vi "main(Test DQMH modules).bak.vi"() -> ()   [LabVIEW 2018, in "Application.lvlib"] (continued)
              frame Disabled {
              }
            }
          }
          event "Test Channel 1": Value Change {
            n428 = event-data() -> ()  [unwired: 1 in, 1 out]
            n429 = Array Subset(array=w1027, index=0, length=6) -> (w1024:refnum<vi>[])
            n430 = for {
              tunnel: w1024 -> [w1036] mode=indexing
              n431 = property class="ColBox"(reference=w1036, "Value"=u32 10000536 ("DRV 1")) -> ()  [unwired: 1 in, 2 out]
            }
            n432 = Build Array("Test Channel 1", "MEAS.AllRelaysOFF") -> (w1031:string[])
            n433 = for {
              tunnel: [w1040] -> w1032 mode=indexing
              tunnel: w1031 -> [w1039] mode=indexing
              tunnel: w1030 -> [w1038]
              n434 = call "App enquece.vi"("command"=w1039, "queue in"=w1038) -> ("error out"=w1040:errorcluster)  [unwired: 8 in, 1 out]
            }
            n435 = Merge Errors(w1034, w1032) -> (w1033:errorcluster)
          }
          event "Test Channel 2": Value Change {
            n436 = event-data() -> ()  [unwired: 1 in, 1 out]
            n437 = Array Subset(array=w1046, index=6, length=6) -> (w1045:refnum<vi>[])
            n438 = for {
              tunnel: w1045 -> [w1057] mode=indexing
              n439 = property class="ColBox"(reference=w1057, "Value"=u32 10000536 ("DRV 1")) -> ()  [unwired: 1 in, 2 out]
            }
            n440 = Build Array("Test Channel 2", "MEAS.AllRelaysOFF") -> (w1052:string[])
            n441 = for {
              tunnel: [w1061] -> w1053 mode=indexing
              tunnel: w1052 -> [w1060] mode=indexing
              tunnel: w1051 -> [w1059]
              n442 = call "App enquece.vi"("command"=w1060, "queue in"=w1059) -> ("error out"=w1061:errorcluster)  [unwired: 8 in, 1 out]
            }
            n443 = Merge Errors(w1055, w1053) -> (w1054:errorcluster)
          }
          event "Test Channel 3": Value Change {
            n444 = event-data() -> ()  [unwired: 1 in, 1 out]
            n445 = Array Subset(array=w1066, index=12, length=6) -> (w1067:refnum<vi>[])
            n446 = for {
              tunnel: w1067 -> [w1078] mode=indexing
              n447 = property class="ColBox"(reference=w1078, "Value"=u32 10000536 ("DRV 1")) -> ()  [unwired: 1 in, 2 out]
            }
            n448 = Build Array("Test Channel 3", "MEAS.AllRelaysOFF") -> (w1073:string[])
            n449 = for {
              tunnel: [w1082] -> w1074 mode=indexing
              tunnel: w1073 -> [w1081] mode=indexing
              tunnel: w1072 -> [w1080]
              n450 = call "App enquece.vi"("command"=w1081, "queue in"=w1080) -> ("error out"=w1082:errorcluster)  [unwired: 8 in, 1 out]
            }
            n451 = Merge Errors(w1076, w1074) -> (w1075:errorcluster)
          }
          event "Test Channel 4": Value Change {
            n452 = event-data() -> ()  [unwired: 1 in, 1 out]
            n453 = Array Subset(array=w1087, index=18, length=6) -> (w1088:refnum<vi>[])
            n454 = for {
              tunnel: w1088 -> [w1099] mode=indexing
              n455 = property class="ColBox"(reference=w1099, "Value"=u32 10000536 ("DRV 1")) -> ()  [unwired: 1 in, 2 out]
            }
            n456 = Build Array("Test Channel 4", "MEAS.AllRelaysOFF") -> (w1094:string[])
            n457 = for {
              tunnel: [w1103] -> w1095 mode=indexing
              tunnel: w1094 -> [w1102] mode=indexing
              tunnel: w1093 -> [w1101]
              n458 = call "App enquece.vi"("command"=w1102, "queue in"=w1101) -> ("error out"=w1103:errorcluster)  [unwired: 8 in, 1 out]
            }
            n459 = Merge Errors(w1097, w1095) -> (w1096:errorcluster)
          }
          event "Test Channel 5": Value Change {
            n460 = event-data() -> ()  [unwired: 1 in, 1 out]
            n461 = Array Subset(array=w1108, index=24, length=6) -> (w1109:refnum<vi>[])
            n462 = for {
              tunnel: w1109 -> [w1120] mode=indexing
              n463 = property class="ColBox"(reference=w1120, "Value"=u32 10000536 ("DRV 1")) -> ()  [unwired: 1 in, 2 out]
            }
            n464 = Build Array("Test Channel 5", "MEAS.AllRelaysOFF") -> (w1115:string[])
            n465 = for {
              tunnel: [w1124] -> w1116 mode=indexing
              tunnel: w1115 -> [w1123] mode=indexing
              tunnel: w1114 -> [w1122]
              n466 = call "App enquece.vi"("command"=w1123, "queue in"=w1122) -> ("error out"=w1124:errorcluster)  [unwired: 8 in, 1 out]
            }
            n467 = Merge Errors(w1118, w1116) -> (w1117:errorcluster)
          }
          event "Test Channel 6": Value Change {
            n468 = event-data() -> ()  [unwired: 1 in, 1 out]
            n469 = Array Subset(array=w1129, index=30, length=6) -> (w1130:refnum<vi>[])
            n470 = for {
              tunnel: w1130 -> [w1141] mode=indexing
              n471 = property class="ColBox"(reference=w1141, "Value"=u32 10000536 ("DRV 1")) -> ()  [unwired: 1 in, 2 out]
            }
            n472 = Build Array("Test Channel 6", "MEAS.AllRelaysOFF") -> (w1136:string[])
            n473 = for {
              tunnel: [w1145] -> w1137 mode=indexing
              tunnel: w1136 -> [w1144] mode=indexing
              tunnel: w1135 -> [w1143]
              n474 = call "App enquece.vi"("command"=w1144, "queue in"=w1143) -> ("error out"=w1145:errorcluster)  [unwired: 8 in, 1 out]
            }
            n475 = Merge Errors(w1139, w1137) -> (w1138:errorcluster)
          }
          event "Test Channel 7": Value Change {
            n476 = event-data() -> ()  [unwired: 1 in, 1 out]
            n477 = Array Subset(array=w1150, index=36, length=6) -> (w1151:refnum<vi>[])
            n478 = for {
              tunnel: w1151 -> [w1162] mode=indexing
              n479 = property class="ColBox"(reference=w1162, "Value"=u32 10000536 ("DRV 1")) -> ()  [unwired: 1 in, 2 out]
            }
            n480 = Build Array("Test Channel 7", "MEAS.AllRelaysOFF") -> (w1158:string[])
            n481 = for {
              tunnel: [w1166] -> w1154 mode=indexing
              tunnel: w1158 -> [w1165] mode=indexing
              tunnel: w1157 -> [w1164]
              n482 = call "App enquece.vi"("command"=w1165, "queue in"=w1164) -> ("error out"=w1166:errorcluster)  [unwired: 8 in, 1 out]
            }
            n483 = Merge Errors(w1160, w1154) -> (w1159:errorcluster)
          }
          event "Test Channel 8": Value Change {
            n484 = event-data() -> ()  [unwired: 1 in, 1 out]
            n485 = Array Subset(array=w1171, index=42, length=6) -> (w1172:refnum<vi>[])
            n486 = for {
              tunnel: w1172 -> [w1183] mode=indexing
              n487 = property class="ColBox"(reference=w1183, "Value"=u32 10000536 ("DRV 1")) -> ()  [unwired: 1 in, 2 out]
            }
            n488 = Build Array("Test Channel 8", "MEAS.AllRelaysOFF") -> (w1178:string[])
            n489 = for {
              tunnel: [w1187] -> w1179 mode=indexing
              tunnel: w1178 -> [w1186] mode=indexing
              tunnel: w1177 -> [w1185]
              n490 = call "App enquece.vi"("command"=w1186, "queue in"=w1185) -> ("error out"=w1187:errorcluster)  [unwired: 8 in, 1 out]
            }
            n491 = Merge Errors(w1181, w1179) -> (w1180:errorcluster)
          }
          event "Test Channel 9": Value Change {
            n492 = event-data() -> ()  [unwired: 1 in, 1 out]
            n493 = Array Subset(array=w1192, index=48, length=6) -> (w1193:refnum<vi>[])
            n494 = for {
              tunnel: w1193 -> [w1204] mode=indexing
              n495 = property class="ColBox"(reference=w1204, "Value"=u32 10000536 ("DRV 1")) -> ()  [unwired: 1 in, 2 out]
            }
            n496 = Build Array("Test Channel 9", "MEAS.AllRelaysOFF") -> (w1199:string[])
            n497 = for {
              tunnel: [w1208] -> w1200 mode=indexing
              tunnel: w1199 -> [w1207] mode=indexing
              tunnel: w1198 -> [w1206]
              n498 = call "App enquece.vi"("command"=w1207, "queue in"=w1206) -> ("error out"=w1208:errorcluster)  [unwired: 8 in, 1 out]
            }
            n499 = Merge Errors(w1202, w1200) -> (w1201:errorcluster)
          }
          event "Test Channel 10": Value Change {
            n500 = event-data() -> ()  [unwired: 1 in, 1 out]
            n501 = Array Subset(array=w1213, index=54, length=6) -> (w1214:refnum<vi>[])
            n502 = for {
              tunnel: w1214 -> [w1225] mode=indexing
              n503 = property class="ColBox"(reference=w1225, "Value"=u32 10000536 ("DRV 1")) -> ()  [unwired: 1 in, 2 out]
            }
            n504 = Build Array("Test Channel 10", "MEAS.AllRelaysOFF") -> (w1220:string[])
            n505 = for {
              tunnel: [w1229] -> w1221 mode=indexing
              tunnel: w1220 -> [w1228] mode=indexing
              tunnel: w1219 -> [w1227]
              n506 = call "App enquece.vi"("command"=w1228, "queue in"=w1227) -> ("error out"=w1229:errorcluster)  [unwired: 8 in, 1 out]
            }
            n507 = Merge Errors(w1223, w1221) -> (w1222:errorcluster)
          }
          event User Event {
            n508 = event-data() -> ("Init?"=w1233:bool)  [unwired: 1 in]
            "DC Measure Module" <- w1233
            "Inst. 1" <- w1233
            n509 = disable-structure shown="LOGGING==TRUE" {
              disable-tunnel: w1236 -> [w1243 _]
              frame condition #0 (active) {
                n510 = Empty String/Path?(string/path=w1243) -> (empty?=w1250:bool)
                n511 = Select(t="Quece timeout", s=w1250, f=w1243) -> (s? t:f=w1248:string)
                n512 = Format Into String(format string=":%s", initial string=w1248, "DMM  Did  it") -> (resulting string=w1245:string)  [unwired: 1 in, 1 out]
                n513 = call "string log (SubVI).vi"("Enum"=enum16{"Init", "Log", "Read"}."Log", "state Name"=w1245) -> ()  [unwired: 8 in, 2 out]
              }
              frame condition #1 {
              }
            }
            n514 = call "FGV Init phase.vi"("Boolean"=w1233) -> ("Init Completed?"=w1232:bool)  [unwired: 9 in, 1 out]
            n515 = case shown="True" w1232 {
              tunnel: w1231 -> [_ w1242]
              frame False {
              }
              frame True {
                n516 = call "App enquece.vi"("command"="INIT.Read DRV code", "queue in"=w1242) -> ()  [unwired: 8 in, 2 out]
              }
            }
            n517 = disable-structure shown="DEBUGGING==TRUE" {
              disable-tunnel: [w1251 w1253] -> w1238
              disable-tunnel: w1237 -> [w1251 w1254]
              frame condition #0 (active) {
              }
              frame condition #1 {
                n518 = call "Show Panel.vi"() -> ("error out"=w1252:errorcluster)  [unwired: 11 in]
                n519 = Merge Errors(w1254, w1252) -> (w1253:errorcluster)
              }
            }
          }
          event User Event {
            n520 = event-data() -> ("Init?"=w1258:bool)  [unwired: 1 in]
            "AC switches Module" <- w1258
            "Inst. 2" <- w1258
            n521 = disable-structure shown="LOGGING==TRUE" {
              disable-tunnel: w1263 -> [w1272 _]
              frame condition #0 (active) {
                n522 = Empty String/Path?(string/path=w1272) -> (empty?=w1279:bool)
                n523 = Select(t="Quece timeout", s=w1279, f=w1272) -> (s? t:f=w1277:string)
                n524 = Format Into String(format string=":%s", initial string=w1277, "MB01  Did  it") -> (resulting string=w1274:string)  [unwired: 1 in, 1 out]
                n525 = call "string log (SubVI).vi"("Enum"=enum16{"Init", "Log", "Read"}."Log", "state Name"=w1274) -> ()  [unwired: 8 in, 2 out]
              }
              frame condition #1 {
              }
            }
            n526 = call "FGV Init phase.vi"("Boolean"=w1258) -> ("Init Completed?"=w1257:bool)  [unwired: 9 in, 1 out]
            n527 = disable-structure shown="DEBUGGING==TRUE" {
              disable-tunnel: [w1268 w1271] -> w1262
              disable-tunnel: w1261 -> [w1268 w1270]
              frame condition #0 (active) {
              }
              frame condition #1 {
                n528 = call "Show Panel.vi"() -> ("error out"=w1269:errorcluster)  [unwired: 11 in]
                n529 = Merge Errors(w1270, w1269) -> (w1271:errorcluster)
              }
            }
            n530 = case shown="True" w1257 {
              tunnel: w1256 -> [_ w1266]
              frame False {
              }
              frame True {
                n531 = call "App enquece.vi"("command"="INIT.Read DRV code", "queue in"=w1266) -> ()  [unwired: 8 in, 2 out]
              }
            }
          }
          event User Event {
            n532 = event-data() -> ("Init?"=w1283:bool)  [unwired: 1 in]
            "DC Switches Module" <- w1283
            "Inst. 3" <- w1283
            n533 = disable-structure shown="LOGGING==TRUE" {
              disable-tunnel: w1286 -> [w1293 _]
              frame condition #0 (active) {
                n534 = Empty String/Path?(string/path=w1293) -> (empty?=w1300:bool)
                n535 = Select(t="Quece timeout", s=w1300, f=w1293) -> (s? t:f=w1298:string)
                n536 = Format Into String(format string=":%s", initial string=w1298, "M054  Did  it") -> (resulting string=w1295:string)  [unwired: 1 in, 1 out]
                n537 = call "string log (SubVI).vi"("Enum"=enum16{"Init", "Log", "Read"}."Log", "state Name"=w1295) -> ()  [unwired: 8 in, 2 out]
              }
              frame condition #1 {
              }
            }
            n538 = call "FGV Init phase.vi"("Boolean"=w1283) -> ("Init Completed?"=w1282:bool)  [unwired: 9 in, 1 out]
            n539 = case shown="True" w1282 {
              tunnel: w1281 -> [_ w1291]
              frame False {
              }
              frame True {
                n540 = call "App enquece.vi"("command"="INIT.Read DRV code", "queue in"=w1291) -> ()  [unwired: 8 in, 2 out]
              }
            }
            n541 = disable-structure shown="DEBUGGING==TRUE" {
              disable-tunnel: w1288 -> [w1301 w1303 w1306]
              disable-tunnel: [w1302 w1303 w1304] -> w1287
              frame condition #0 (active) {
                n542 = Merge Errors(w1301) -> (w1302:errorcluster)
              }
              frame condition #1 {
              }
              frame condition #2 {
                n543 = call "Show Panel.vi"() -> ("error out"=w1305:errorcluster)  [unwired: 11 in]
                n544 = Merge Errors(w1306, w1305) -> (w1304:errorcluster)
              }
            }
          }
        }
      }
      frame "Apps.AutoMode" {
        n545 = disable-structure shown="Disabled" {
          frame Disabled {
            n546 = local write "Auto/Man"(TRUE) -> ()
          }
          frame Enabled {
          }
        }
      }
      frame "Apps.WaitingForTrigger" {
        n547 = call "App enquece.vi"("command"="MEAS.Read TRIGGER", "queue in"=w1321) -> ("error out"=w1319:errorcluster)  [unwired: 8 in, 1 out]
        n548 = Merge Errors(w1317, w1319) -> (w1318:errorcluster)
      }
      frame "Apps.UpdateStatus" {
        n549 = disable-structure shown="LOGGING==TRUE" {
          disable-tunnel: w1329 -> [w1342 _]
          frame condition #0 (active) {
            n550 = Empty String/Path?(string/path=w1342) -> (empty?=w1345:bool)
            n551 = Select(t="Quece timeout", s=w1345, f=w1342) -> (s? t:f=w1341:string)
            n552 = call "string log (SubVI).vi"("Enum"=enum16{"Init", "Log", "Read"}."Log", "state Name"=w1341) -> ()  [unwired: 8 in, 2 out]
          }
          frame condition #1 {
          }
        }
        n553 = call "App enquece.vi"("command"="Apps.WaitForEvent", "queue in"=w1337) -> ("error out"=w1334:errorcluster)  [unwired: 8 in, 1 out]
        n554 = Merge Errors(w1330, w1334) -> (w1331:errorcluster)
      }
      frame "Apps.UI Update" {
        n555 = disable-structure shown="LOGGING==TRUE" {
          disable-tunnel: w1349 -> [w1397 _]
          frame condition #0 (active) {
            n556 = Empty String/Path?(string/path=w1397) -> (empty?=w1400:bool)
            n557 = Select(t="Quece timeout", s=w1400, f=w1397) -> (s? t:f=w1396:string)
            n558 = call "string log (SubVI).vi"("Enum"=enum16{"Init", "Log", "Read"}."Log", "state Name"=w1396) -> ()  [unwired: 8 in, 2 out]
          }
          frame condition #1 {
          }
        }
        n559 = Variant To Data(type="", Variant=w1347) -> (data=w1346:string)  [unwired: 1 in, 1 out]
        n560 = case shown="\"A\"" w1346 {
          tunnel: [w1370 w1378] -> w1355
          tunnel: w1353 -> [w1368 w1379]
          tunnel: w1352 -> [w1365 w1380]
          frame "", Default {
            w1362 = 6 ("length")
            n561 = call "FGV Driver Data.vi"("DUT channel (1-11)"=w1365, "FGV enum(Read)"=FGV_DRV_data."Process" ("FGV DRV data enum")) -> ("60 DRV data"=w1363:T17[])  [unwired: 6 in, 3 out]
            n562 = Decrement(x=w1365) -> (x-1=w1366:i32)
            n563 = Multiply(x=w1366, y=w1362) -> (x*y=w1364:i32)
            n564 = Array Subset(array=w1363, index=w1364, length=w1362) -> (w1361:T17[])
            n565 = Array Subset(array=w1368, index=w1364, length=w1362) -> (w1367:refnum<vi>[])
            n566 = for {
              tunnel: w1367 -> [w1373] mode=indexing
              tunnel: w1361 -> [w1372] mode=indexing
              tunnel: [w1371] -> w1370 mode=indexing
              n567 = Unbundle By Name(w1372) -> ("DRV Fail/Pass (T)"=w1376:bool)
              n568 = Select(t=u32 16711686 ("DRV 1"), s=w1376, f=u32 65309 ("DRV 1")) -> (s? t:f=w1377:u32)
              n569 = property class="ColBox"(reference=w1373, "Value"=w1377) -> (error out=w1371:errorcluster)  [unwired: 1 in, 1 out]
            }
          }
          frame "A" {
            w1381 = 2
            n570 = call "FGV Driver Data.vi"("DUT channel (1-11)"=w1380, "FGV enum(Read)"=FGV_DRV_data."Process" ("FGV DRV data enum")) -> ("60 DRV data"=w1384:T17[])  [unwired: 6 in, 3 out]
            n571 = Decrement(x=w1380) -> (x-1=w1386:i32)
            n572 = Multiply(x=w1386, y=6 ("length")) -> (x*y=w1385:i32)
            n573 = Array Subset(array=w1384, index=w1385, length=w1381) -> (w1382:T17[])
            n574 = Array Subset(array=w1379, index=w1385, length=w1381) -> (w1387:refnum<vi>[])
            n575 = for {
              tunnel: w1387 -> [w1391] mode=indexing
              tunnel: w1382 -> [w1390] mode=indexing
              tunnel: [w1389] -> w1378 mode=indexing
              n576 = Unbundle By Name(w1390) -> ("DRV Fail/Pass (T)"=w1394:bool)
              n577 = Select(t=u32 16711686 ("DRV 1"), s=w1394, f=u32 65309 ("DRV 1")) -> (s? t:f=w1395:u32)
              n578 = property class="ColBox"(reference=w1391, "Value"=w1395) -> (error out=w1389:errorcluster)  [unwired: 1 in, 1 out]
            }
          }
        }
        n579 = Merge Errors(w1356, w1355) -> (w1357:errorcluster)
      }
      frame "Apps.UI Update 1" {
        n580 = disable-structure shown="LOGGING==TRUE" {
          disable-tunnel: w1415 -> [w1423 _]
          frame condition #0 (active) {
            n581 = Empty String/Path?(string/path=w1423) -> (empty?=w1426:bool)
            n582 = Select(t="Quece timeout", s=w1426, f=w1423) -> (s? t:f=w1422:string)
            n583 = call "string log (SubVI).vi"("Enum"=enum16{"Init", "Log", "Read"}."Log", "state Name"=w1422) -> ()  [unwired: 8 in, 2 out]
          }
          frame condition #1 {
          }
        }
        n584 = call "FGV Driver Data.vi"("DUT channel (1-11)"=w1413, "FGV enum(Read)"=FGV_DRV_data."Process" ("FGV DRV data enum")) -> ("60 DRV data"=w1406:T17[])  [unwired: 6 in, 3 out]
        n585 = Decrement(x=w1401) -> (x-1=w1402:i32)
        n586 = Index Array(array=w1406, index=w1402) -> (element=w1405:T17)
        n587 = Index Array(array=w1407, index=w1402) -> (element=w1404:refnum<vi>)
        n588 = Unbundle By Name(w1405) -> ("DRV Fail/Pass (T)"=w1403:bool)
        n589 = Select(t=u32 16711686 ("DRV 1"), s=w1403, f=u32 65309 ("DRV 1")) -> (s? t:f=w1410:u32)
        n590 = property class="ColBox"(reference=w1404, "Value"=w1410) -> (error out=w1416:errorcluster)  [unwired: 1 in, 1 out]
        n591 = Merge Errors(w1417, w1416) -> (w1418:errorcluster)
      }
      frame "Apps.UI Update 2" {
        n592 = disable-structure shown="Enabled" {
          disable-tunnel: w1431 -> [w1459 _]
          disable-tunnel: [w1457 _] -> w1430
          frame Enabled {
            n593 = call "App enquece.vi"("command"="Apps.AutoMode", "queue in"=w1459) -> ("error out"=w1457:errorcluster)  [unwired: 8 in, 1 out]
          }
          frame Disabled {
          }
        }
        n594 = disable-structure shown="LOGGING==TRUE" {
          disable-tunnel: w1440 -> [w1477 _]
          frame condition #0 (active) {
            n595 = Empty String/Path?(string/path=w1477) -> (empty?=w1480:bool)
            n596 = Select(t="Quece timeout", s=w1480, f=w1477) -> (s? t:f=w1476:string)
            n597 = call "string log (SubVI).vi"("Enum"=enum16{"Init", "Log", "Read"}."Log", "state Name"=w1476) -> ()  [unwired: 8 in, 2 out]
          }
          frame condition #1 {
          }
        }
        n598 = local read "Enum"() -> (w1435:T1)
        n599 = call "FGV Driver Data.vi"("error in (no error)"=w1430, "FGV enum(Read)"=FGV_DRV_data."Process" ("FGV DRV data enum")) -> ("error out"=w1439:errorcluster, "60 DRV data"=w1436:T17[])  [unwired: 6 in, 2 out]
        n600 = case shown="\"00037845(M26)\"" w1435 {
          tunnel: w1436 -> [w1467 w1469 w1471 w1475]
          tunnel: [w1466 w1468 w1471 w1474] -> w1428
          frame "Fixxed", Default {
            n601 = Array Subset(array=w1467, length=41) -> (w1466:T17[])  [unwired: 1 in]
          }
          frame "Pinpoint_JIG" {
            n602 = Array Subset(array=w1469, index=42) -> (w1468:T17[])  [unwired: 1 in]
          }
          frame "All DRV" {
          }
          frame "00037845(M26)" {
            n603 = Array Subset(array=w1475, index=42, length=14) -> (w1474:T17[])
          }
        }
        n604 = for {
          tunnel: w1428 -> [w1482] mode=indexing
          tunnel: [w1481] -> w1446 mode=indexing
          n605 = Unbundle By Name(w1482) -> ("DRV Fail/Pass (T)"=w1481:bool)
        }
        n606 = Or Array Elements(Boolean array=w1446) -> (logical OR=w1444:bool)
        n607 = control-ref of="DRV 61"() -> (w1445:refnum<vi>)
        n608 = Select(t=u32 16711680 ("DRV 1"), s=w1444, f=u32 6618880 ("DRV 1")) -> (s? t:f=w1441:u32)
        n609 = property class="ColBox"(reference=w1445, error in=w1439, "Value"=w1441) -> (error out=w1438:errorcluster)  [unwired: 1 out]
        n610 = case shown="True" "Log report" {
          tunnel: w1428 -> [_ w1455]
          tunnel: w1427 -> [_ w1456]
          frame False {
          }
          frame True {
            n611 = To Variant(anything=w1455) -> (Variant=w1454:variant)
            n612 = Enqueue Element(queue=w1456, element=w1454) -> ()  [unwired: 2 in, 3 out]
          }
        }
        n613 = Merge Errors(w1453, w1438) -> (w1432:errorcluster)
        n614 = disable-structure shown="NO_HARDWARE==TRUE" {
          disable-tunnel: [w1462 w1464] -> w1433
          disable-tunnel: w1432 -> [w1462 w1464]
          frame condition #0 (active) {
            n615 = Wait (ms)(milliseconds to wait=u32 2000) -> ()  [unwired: 1 out]
          }
          frame condition #1 {
          }
        }
        n616 = disable-structure shown="Disabled" {
          frame Disabled {
            n617 = local read "Auto/Man"() -> (w1460:bool)
            n618 = case shown="True" w1460 {
              frame False {
              }
              frame True {
                n619 = property on="Test" class="Bool"("Val(Sgnl)"=TRUE ("Value (Signaling)")) -> ()  [unwired: 2 in, 2 out]
              }
            }
          }
          frame Enabled {
          }
        }
      }
      frame "Apps.UI Update SC" {
        w1488 = "All Shorted Circuits"
        n620 = disable-structure shown="LOGGING==TRUE" {
          disable-tunnel: w1494 -> [w1527 _]
          frame condition #0 (active) {
            n621 = Empty String/Path?(string/path=w1527) -> (empty?=w1530:bool)
            n622 = Select(t="Quece timeout", s=w1530, f=w1527) -> (s? t:f=w1526:string)
            n623 = call "string log (SubVI).vi"("Enum"=enum16{"Init", "Log", "Read"}."Log", "state Name"=w1526) -> ()  [unwired: 8 in, 2 out]
          }
          frame condition #1 {
          }
        }
        n624 = local read "Enum"() -> (w1487:T1)
        n625 = call "FGV Driver Data.vi"("FGV enum(Read)"=FGV_DRV_data."Read" ("FGV DRV data enum")) -> ("60 DRV data"=w1484:T17[])  [unwired: 7 in, 3 out]
        n626 = case shown="\"00037845(M26)\"" w1487 {
          tunnel: w1486 -> [w1507 w1512 w1514 w1519]
          tunnel: [w1506 w1508 w1514 w1517] -> w1485
          tunnel: w1484 -> [w1505 w1511 w1513 w1518]
          tunnel: [w1503 w1510 w1513 w1516] -> w1483
          frame "Fixxed", Default {
            w1504 = 42 ("length")
            n627 = Array Subset(array=w1505, length=w1504) -> (w1503:T17[])  [unwired: 1 in]
            n628 = Array Subset(array=w1507, length=w1504) -> (w1506:refnum<vi>[])  [unwired: 1 in]
          }
          frame "Pinpoint_JIG" {
            w1509 = 42 ("length")
            n629 = Array Subset(array=w1512, index=w1509) -> (w1508:refnum<vi>[])  [unwired: 1 in]
            n630 = Array Subset(array=w1511, index=w1509) -> (w1510:T17[])  [unwired: 1 in]
          }
          frame "All DRV" {
          }
          frame "00037845(M26)" {
            w1515 = 14 ("length")
            w1520 = 42 ("length")
            n631 = Array Subset(array=w1519, index=w1520, length=w1515) -> (w1517:refnum<vi>[])
            n632 = Array Subset(array=w1518, index=w1520, length=w1515) -> (w1516:T17[])
          }
        }
        n633 = for {
          tunnel: w1483 -> [w1537] mode=indexing
          tunnel: w1485 -> [w1532] mode=indexing
          tunnel: [w1531] -> w1492 mode=indexing
          n634 = Unbundle By Name(w1537) -> ("Shorted Circuit"=w1533:bool)
          n635 = Select(t=u32 16711680 ("DRV 1"), s=w1533, f=u32 6618880 ("DRV 1")) -> (s? t:f=w1536:u32)
          n636 = property class="ColBox"(reference=w1532, "Value"=w1536) -> (error out=w1531:errorcluster)  [unwired: 1 in, 1 out]
        }
        n637 = Merge Errors(w1492) -> (w1491:errorcluster)
        n638 = flat-sequence {
          tunnel: w1491 -> [w1522]
          tunnel: [w1522] -> w1490
          tunnel: w1490 -> [w1524]
          tunnel: [w1525] -> w1489
          tunnel: w1486 -> [w1523]
          frame #0 {
            n639 = Wait (ms)(milliseconds to wait=u32 1500) -> ()  [unwired: 1 out]
          }
          frame #1 {
            n640 = call "reset DRV UI (SubVI).vi"("error in (no error)"=w1524, "Ref  in"=w1523) -> ("error out"=w1525:errorcluster)  [unwired: 8 in, 1 out]
          }
        }
        n641 = Merge Errors(w1502, w1489) -> (w1493:errorcluster)
        n642 = local write "Progress"(w1488) -> ()
      }
      frame "Timer Start" {
        n643 = flat-sequence {
          tunnel: [u32 0 ("time elased(ms)")] -> w1538
          frame #0 {
            n644 = call "FGV milisec (subVI).vi"() -> ()  [unwired: 11 in, 1 out]
          }
        }
        n645 = local write "time elased(ms)"(w1538) -> ()
      }
      frame "Timer Stop" {
        n646 = flat-sequence {
          tunnel: [w1559] -> w1548
          tunnel: w1549 -> [w1559]
          tunnel: [w1558] -> w1550
          frame #0 {
            n647 = call "FGV milisec (subVI).vi"() -> ("Elased Time (ms)"=w1558:u32)  [unwired: 11 in]
          }
        }
        "time elased(ms)" <- w1550
      }
      frame "WaitFor" {
        n648 = Variant To Data(type=u32 0, Variant=w1560) -> ()  [unwired: 1 in, 2 out]
        n649 = Wait (ms)(milliseconds to wait="milliseconds to wait") -> ()  [unwired: 1 out]
      }
      frame "Apps.Exit" {
        w1575 = TRUE
        n650 = disable-structure shown="LOGGING==TRUE" {
          disable-tunnel: w1572 -> [w1590 _]
          frame condition #0 (active) {
            n651 = Empty String/Path?(string/path=w1590) -> (empty?=w1593:bool)
            n652 = Select(t="Quece timeout", s=w1593, f=w1590) -> (s? t:f=w1589:string)
            n653 = call "string log (SubVI).vi"("Enum"=enum16{"Init", "Log", "Read"}."Log", "state Name"=w1589) -> ()  [unwired: 8 in, 2 out]
          }
          frame condition #1 {
          }
        }
        n654 = call "Application Name--constant.vi"() -> ("Application Name"=w1576:string)  [unwired: 11 in]
        n655 = call "Stop Module.vi"("Wait for Module to stop? (F)"=w1575, "Origin"=w1576, "Module ID"=-1) -> ("error out"=w1578:errorcluster)  [unwired: 8 in]
        n656 = call "Stop Module.vi"("Wait for Module to Stop? (F)"=w1575, "Origin"=w1576) -> ("error out"=w1584:errorcluster)  [unwired: 9 in]
        n657 = call "Stop Module.vi"("Wait for Module to Stop? (F)"=w1575, "Origin"=w1576) -> ("error out"=w1583:errorcluster)  [unwired: 9 in]
        n658 = call "Stop Module.vi"("Wait for Module to Stop? (F)"=w1575, "Origin"=w1576) -> ("error out"=w1582:errorcluster)  [unwired: 9 in]
        n659 = Merge Errors(w1580, w1584, w1583, w1582, w1578) -> (w1581:errorcluster)
      }
      frame "Apps.Error Handler" {
        w1602 = TRUE  # Priority Enquece
        n660 = disable-structure shown="LOGGING==TRUE" {
          disable-tunnel: w1595 -> [w1611 _]
          frame condition #0 (active) {
            n661 = Empty String/Path?(string/path=w1611) -> (empty?=w1614:bool)
            n662 = Select(t="Quece timeout", s=w1614, f=w1611) -> (s? t:f=w1610:string)
            n663 = call "string log (SubVI).vi"("Enum"=enum16{"Init", "Log", "Read"}."Log", "state Name"=w1610) -> ()  [unwired: 8 in, 2 out]
          }
          frame condition #1 {
          }
        }
        n664 = call <vilib>:"Simple Error Handler.vi"("error in (no error)"=w1609) -> ("error out"=w1604:errorcluster)  [unwired: 4 in, 4 out]
        n665 = flat-sequence {
          tunnel: w1604 -> [_]
          tunnel: [w1615] -> w1596
          frame #0 {
            n666 = xnode "Error Ring"() -> ("error out"=w1615:errorcluster)
          }
        }
        n667 = call "App enquece.vi"("Priority Enquece"=w1602, "command"="Apps.Exit", "queue in"=w1603) -> ("error out"=w1601:errorcluster)  [unwired: 7 in, 1 out]
        n668 = Merge Errors(w1596, w1601) -> (w1597:errorcluster)
      }
      frame "INIT.Init FGV" {
        n669 = call "FGV_HoldingRegs.vi"("FGV_enum"=FGV_enum."Init FGV") -> ("error out"=w1624:errorcluster)  [unwired: 8 in, 2 out]
        n670 = call "string log (SubVI).vi"("error in (no error)"=w1624, "Enum"=enum16{"Init", "Log", "Read"}."Init") -> ("error out"=w1625:errorcluster)  [unwired: 8 in, 1 out]
        n671 = local write "EMIC connected"(bool[] [FALSE, FALSE, FALSE, FALSE, FALSE, FALSE] ("Array")) -> ()
        n672 = local write "Auto/Man"(FALSE) -> ()
        n673 = call "FGV Driver Data.vi"("error in (no error)"=w1625, "FGV enum(Read)"=FGV_DRV_data."Init" ("FGV DRV data enum")) -> ("error out"=w1622:errorcluster)  [unwired: 6 in, 3 out]
        n674 = call "FGV Init phase.vi"("error in (no error)"=w1622, "FGV Enum"=enum16{"Init", "Check"}."Init") -> ("error out"=w1621:errorcluster)  [unwired: 8 in, 1 out]
        n675 = Initialize Array(FALSE, 6 ("dimension size"), 10 ("dimension size")) -> (w1620:bool[][])
        n676 = local write "Short DRV"(w1620) -> ()
        n677 = Merge Errors(w1639, w1621) -> (w1628:errorcluster)
      }
      frame "INIT.Read HW config" {
        n678 = disable-structure shown="LOGGING==TRUE" {
          disable-tunnel: w1646 -> [w1682 _]
          frame condition #0 (active) {
            n679 = Empty String/Path?(string/path=w1682) -> (empty?=w1685:bool)
            n680 = Select(t="Quece timeout", s=w1685, f=w1682) -> (s? t:f=w1681:string)
            n681 = call "string log (SubVI).vi"("Enum"=enum16{"Init", "Log", "Read"}."Log", "state Name"=w1681) -> ()  [unwired: 8 in, 2 out]
          }
          frame condition #1 {
          }
        }
        n682 = disable-structure shown="Default" {
          disable-tunnel: ["Development" ("version") "Released"] -> w1645
          frame condition #0 (active) {
          }
          frame condition #1 {
          }
        }
        "version" <- w1645
        n683 = call <vilib>:"Application Directory.vi"() -> ("Application Directory"=w1641:path)
        n684 = Build Path(base path=w1641, name or relative path="config") -> (appended path=w1640:path)
        n685 = call "HW Config.vi"("start path"=w1640) -> ("error out"=w1647:errorcluster, "HW config 2"=w1654:T9)  [unwired: 9 in]
        n686 = Bundle By Name(cluster=w1655, "HW config 2"=w1654) -> (w1653:cluster{"HW config 2":T9})
        n687 = disable-structure shown="Enabled" {
          disable-tunnel: [w1665 w1680] -> w1648
          disable-tunnel: w1647 -> [w1664 w1680]
          disable-tunnel: w1643 -> [w1663 _]
          frame Enabled {
            n688 = invoke class="VI" method="FP.Open"(error in=w1664, "State"=T18."Minimized") -> (error out=w1666:errorcluster)  [unwired: 3 in, 4 out]
            n689 = call "Login.vi"("error in (no error)"=w1666) -> ("error out"=w1668:errorcluster, "Login Successed"=w1669:bool, "UserName"=w1662:string)  [unwired: 8 in]
            n690 = call "FGV _Operator Name.vi"("Enum"=enum16{"Write", "Read"}."Write", "Operator Name in"=w1662) -> ()  [unwired: 9 in, 1 out]
            n691 = case shown="True" w1669 {
              tunnel: w1663 -> [w1676 _]
              tunnel: w1668 -> [w1673 w1678]
              tunnel: [w1672 w1679] -> w1665
              frame False {
                n692 = call "string log (SubVI).vi"("Enum"=enum16{"Init", "Log", "Read"}."Init") -> ("error out"=w1670:errorcluster)  [unwired: 9 in, 1 out]
                n693 = call "App enquece.vi"("Priority Enquece"=TRUE, "error in (no error)"=w1673, "command"="Apps.Exit", "queue in"=w1676) -> ("error out"=w1672:errorcluster)  [unwired: 6 in, 1 out]
                n694 = call "inst.InitialiseFGV.vi"("error in (no error)"=w1670) -> ()  [unwired: 10 in, 1 out]
              }
              frame True {
                n695 = invoke class="VI" method="FP.Open"(error in=w1678, "State"=T18."Standard") -> (error out=w1679:errorcluster)  [unwired: 3 in, 4 out]
              }
            }
          }
          frame Disabled {
          }
        }
        n696 = Merge Errors(w1658, w1648) -> (w1649:errorcluster)
      }
      frame "INIT.Read DRV code" {
        w1711 = u8 2 items=["SLOW", "MID", "FAST"] ("Detector Rate")
        # "Convert from [mA] to [A]"
        n697 = disable-structure shown="LOGGING==TRUE" {
          disable-tunnel: w1719 -> [w1729 _]
          frame condition #0 (active) {
            n698 = Empty String/Path?(string/path=w1729) -> (empty?=w1732:bool)
            n699 = Select(t="Quece timeout", s=w1732, f=w1729) -> (s? t:f=w1728:string)
            n700 = call "string log (SubVI).vi"("Enum"=enum16{"Init", "Log", "Read"}."Log", "state Name"=w1728) -> ()  [unwired: 8 in, 2 out]
          }
          frame condition #1 {
          }
        }
        n701 = invoke class="VI" method="FP.Open"("State"=T18."Hidden") -> (error out=w1696:errorcluster)  [unwired: 4 in, 4 out]
        n702 = call "ReadDriverParameters.vi"("error in (no error)"=w1696) -> ("error out"=w1694:errorcluster, "DRV stand"=w1702:T2)  [unwired: 9 in]
        n703 = invoke class="VI" method="FP.Open"(error in=w1694, "State"=T18."Standard") -> (error out=w1698:errorcluster)  [unwired: 3 in, 4 out]
        n704 = Merge Errors(w1720, w1698) -> (w1721:errorcluster)
        n705 = call "FGV DRV stand.vi"("Enum"=enum16{"Write", "Read"}."Write", "DRV stand  in"=w1702) -> ("DRV stand out"=w1699:T2)  [unwired: 9 in]
        "DRV stand" <- w1699
        n706 = Unbundle By Name(w1699) -> ("SAP ID"=w1687:string, "Name"=w1688:string)
        "SAP ID" <- w1687
        "Name" <- w1688
        n707 = Unbundle By Name(w1702) -> ("DC characteristics.Voltage.Max"=w1693:dbl, "DC characteristics.Current.Max"=w1718:dbl)
        n708 = call "FGV SapID & Name.vi"("Enum"=enum16{"Read", "Write"}."Write", "Name"=w1688, "SAP ID"=w1687) -> ()  [unwired: 6 in, 3 out]
        n709 = Divide(x=w1718, y=1000.0) -> (x/y=w1690:dbl)
        n710 = Greater?(x=w1690, y=0.5) -> (0:w1691:bool)
        n711 = Bundle By Name(cluster=T19 {"DMM config cluster"={"DCV range"=0.0, "DCI range"=0.0, "Detector Rate"=0}, "mux2-1(DMM I) encode"=enum."DMM I (0.5)"} ("DMM all config"), "DMM config cluster.DCV range"=w1693, "DMM config cluster.DCI range"=w1690, "DMM config cluster.Detector Rate"=w1711) -> (w1715:T19)
        n712 = Select(t=enum16{"DMM I (0.5)", "DMM I (12)"}."DMM I (12)" ("mux2-1(DMM I) encode 2"), s=w1691, f=enum16{"DMM I (0.5)", "DMM I (12)"}."DMM I (0.5)" ("mux2-1(DMM I) encode 2")) -> (s? t:f=w1706:enum16{"DMM I (0.5)", "DMM I (12)"})
        n713 = To Variant(anything=w1715) -> (Variant=w1714:variant)
        n714 = To Variant(anything=w1706) -> (Variant=w1708:variant)
        n715 = call "App enquece.vi"("command data"=w1714, "command"="MEAS.Set DMM config", "queue in"=w1712) -> ("error out"=w1703:errorcluster, "Queue out"=w1707:refnum<queue>)  [unwired: 7 in]
        n716 = call "App enquece.vi"("error in (no error)"=w1703, "command data"=w1708, "command"="MEAS.Sel Input Current", "queue in"=w1707) -> ("error out"=w1689:errorcluster)  [unwired: 6 in, 1 out]
        n717 = Merge Errors(w1721, w1689) -> (w1710:errorcluster)
      }
      frame "INIT.Call DMM module" {
        n718 = disable-structure shown="LOGGING==TRUE" {
          disable-tunnel: w1734 -> [w1752 _]
          frame condition #0 (active) {
            n719 = Empty String/Path?(string/path=w1752) -> (empty?=w1755:bool)
            n720 = Select(t="Quece timeout", s=w1755, f=w1752) -> (s? t:f=w1751:string)
            n721 = call "string log (SubVI).vi"("Enum"=enum16{"Init", "Log", "Read"}."Log", "state Name"=w1751) -> ()  [unwired: 8 in, 2 out]
          }
          frame condition #1 {
          }
        }
        n722 = Unbundle By Name(w1745) -> ("HW config 2.DMM"=w1744:string)
        n723 = Type Cast(type=refnum<visa-resource-name> refnum ("VISA resource name 2"), x=w1744) -> (*(type *) &x=w1742:refnum<visa-resource-name>)
        n724 = call "Start Module.vi"("VISA resource name 2"=w1742) -> ("error out"=w1747:errorcluster, "Wait for Event Sync?"=w1741:bool, "DMM Module Broadcast Events"=w1740:T15)  [unwired: 7 in, 1 out]
        n725 = register-events(reference=w1748, w1740) -> (reference out=w1749:refnum<event-registration>)  [unwired: 5 in, 1 out]
        n726 = call "Synchronize Module Events.vi"("error in"=w1747, "Wait for Event Sync?"=w1741) -> ("error out"=w1746:errorcluster)  [unwired: 9 in]
        n727 = Merge Errors(w1735, w1746) -> (w1736:errorcluster)
      }
      frame "INIT.Call MUX module" {
        n728 = disable-structure shown="LOGGING==TRUE" {
          disable-tunnel: w1757 -> [w1775 _]
          frame condition #0 (active) {
            n729 = Empty String/Path?(string/path=w1775) -> (empty?=w1778:bool)
            n730 = Select(t="Quece timeout", s=w1778, f=w1775) -> (s? t:f=w1774:string)
            n731 = call "string log (SubVI).vi"("Enum"=enum16{"Init", "Log", "Read"}."Log", "state Name"=w1774) -> ()  [unwired: 8 in, 2 out]
          }
          frame condition #1 {
          }
        }
        n732 = Unbundle By Name(w1769) -> ("HW config 2.mux"=w1768:string)
        n733 = Type Cast(type=refnum<visa-resource-name> refnum ("VISA resource name"), x=w1768) -> (*(type *) &x=w1767:refnum<visa-resource-name>)
        n734 = call "Start Module.vi"("VISA resource name"=w1767) -> ("error out"=w1770:errorcluster, "Wait for Event Sync?"=w1764:bool, "Switches Module Broadcast Events"=w1765:T13)  [unwired: 7 in, 1 out]
        n735 = register-events(reference=w1771, w1765) -> (reference out=w1772:refnum<event-registration>)  [unwired: 5 in, 1 out]
        n736 = call "Synchronize Module Events.vi"("error in"=w1770, "Wait for Event Sync?"=w1764) -> ("error out"=w1763:errorcluster)  [unwired: 9 in]
        n737 = Merge Errors(w1758, w1763) -> (w1759:errorcluster)
      }
      frame "INIT.Call DEMUX module" {
        n738 = disable-structure shown="LOGGING==TRUE" {
          disable-tunnel: w1780 -> [w1798 _]
          frame condition #0 (active) {
            n739 = Empty String/Path?(string/path=w1798) -> (empty?=w1801:bool)
            n740 = Select(t="Quece timeout", s=w1801, f=w1798) -> (s? t:f=w1797:string)
            n741 = call "string log (SubVI).vi"("Enum"=enum16{"Init", "Log", "Read"}."Log", "state Name"=w1797) -> ()  [unwired: 8 in, 2 out]
          }
          frame condition #1 {
          }
        }
        n742 = Unbundle By Name(w1791) -> ("HW config 2.demux"=w1790:string)
        n743 = Type Cast(type=refnum<visa-resource-name> refnum ("COMport name"), x=w1790) -> (*(type *) &x=w1789:refnum<visa-resource-name>)
        n744 = call "Start Module.vi"("COMport name"=w1789) -> ("error out"=w1792:errorcluster, "Wait for Event Sync?"=w1793:bool, "MB 01 switches Module Broadcast Events"=w1787:T14)  [unwired: 7 in, 1 out]
        n745 = call "Synchronize Module Events.vi"("error in"=w1792, "Wait for Event Sync?"=w1793) -> ("error out"=w1786:errorcluster)  [unwired: 9 in]
        n746 = register-events(reference=w1794, w1787) -> (reference out=w1795:refnum<event-registration>)  [unwired: 5 in, 1 out]
        n747 = Merge Errors(w1781, w1786) -> (w1782:errorcluster)
      }
      frame "INIT.Call EMIC modules" {
        n748 = disable-structure shown="LOGGING==TRUE" {
          disable-tunnel: w1805 -> [w1822 _]
          frame condition #0 (active) {
            n749 = Empty String/Path?(string/path=w1822) -> (empty?=w1825:bool)
            n750 = Select(t="Quece timeout", s=w1825, f=w1822) -> (s? t:f=w1821:string)
            n751 = call "string log (SubVI).vi"("Enum"=enum16{"Init", "Log", "Read"}."Log", "state Name"=w1821) -> ()  [unwired: 8 in, 2 out]
          }
          frame condition #1 {
          }
        }
        n752 = Unbundle By Name(w1812) -> ("HW config 2.eMIC1"=w1819:string, "HW config 2.eMIC2"=w1818:string, "HW config 2.eMIC3"=w1817:string, "HW config 2.eMIC4"=w1816:string, "HW config 2.eMIC5"=w1815:string, "HW config 2.eMIC6"=w1814:string)
        n753 = Build Array(w1819, w1818, w1817, w1816, w1815, w1814) -> (w1803:string[])
        n754 = for {
          shift-right: [w1835] -> w1811
          shift-left: w1813 -> [w1833]
          tunnel: w1803 -> [w1834] mode=indexing
          tunnel: [w1827] -> w1809 mode=indexing
          n755 = Type Cast(type=refnum<visa-resource-name> refnum ("VISA resource name"), x=w1834) -> (*(type *) &x=w1831:refnum<visa-resource-name>)
          n756 = call "Start Module.vi"("VISA resource name"=w1831) -> ("error out"=w1828:errorcluster, "Wait for Event Sync?"=w1826:bool, "CE14_v2 Broadcast Events"=w1830:T12, "Module ID"=w1829:i32)  [unwired: 7 in]
          n757 = register-events(reference=w1833, w1830) -> (reference out=w1835:refnum<event-registration>)  [unwired: 5 in, 1 out]
          n758 = call "Synchronize Module Events.vi"("error in"=w1828, "Wait for Event Sync?"=w1826, "Module ID in"=w1829) -> ("error out"=w1827:errorcluster)  [unwired: 7 in, 1 out]
        }
        n759 = Merge Errors(w1806, w1809) -> (w1804:errorcluster)
      }
      frame "INIT.Open COM DMM" {
        n760 = disable-structure shown="LOGGING==TRUE" {
          disable-tunnel: w1839 -> [w1851 _]
          frame condition #0 (active) {
            n761 = Empty String/Path?(string/path=w1851) -> (empty?=w1854:bool)
            n762 = Select(t="Quece timeout", s=w1854, f=w1851) -> (s? t:f=w1850:string)
            n763 = call "string log (SubVI).vi"("Enum"=enum16{"Init", "Log", "Read"}."Log", "state Name"=w1850) -> ()  [unwired: 8 in, 2 out]
          }
          frame condition #1 {
          }
        }
        n764 = call "DMM connect and reset.vi"() -> ("error out"=w1843:errorcluster)  [unwired: 11 in]
        n765 = Merge Errors(w1840, w1843) -> (w1837:errorcluster)
        n766 = flat-sequence {
          tunnel: [w1849] -> w1838
          tunnel: w1837 -> [w1849]
          frame #0 {
            n767 = Wait (ms)(milliseconds to wait=u32 70) -> ()  [unwired: 1 out]
          }
        }
      }
      frame "INIT.Open COM MUX" {
        n768 = disable-structure shown="LOGGING==TRUE" {
          disable-tunnel: w1858 -> [w1870 _]
          frame condition #0 (active) {
            n769 = Empty String/Path?(string/path=w1870) -> (empty?=w1873:bool)
            n770 = Select(t="Quece timeout", s=w1873, f=w1870) -> (s? t:f=w1869:string)
            n771 = call "string log (SubVI).vi"("Enum"=enum16{"Init", "Log", "Read"}."Log", "state Name"=w1869) -> ()  [unwired: 8 in, 2 out]
          }
          frame condition #1 {
          }
        }
        n772 = call "inst.Open.vi"() -> ("error out"=w1864:errorcluster)  [unwired: 11 in]
        n773 = Merge Errors(w1859, w1864) -> (w1856:errorcluster)
        n774 = flat-sequence {
          tunnel: [w1868] -> w1857
          tunnel: w1856 -> [w1868]
          frame #0 {
            n775 = Wait (ms)(milliseconds to wait=u32 70) -> ()  [unwired: 1 out]
          }
        }
      }
      frame "INIT.Open COM DEMUX" {
        n776 = disable-structure shown="LOGGING==TRUE" {
          disable-tunnel: w1877 -> [w1889 _]
          frame condition #0 (active) {
            n777 = Empty String/Path?(string/path=w1889) -> (empty?=w1892:bool)
            n778 = Select(t="Quece timeout", s=w1892, f=w1889) -> (s? t:f=w1888:string)
            n779 = call "string log (SubVI).vi"("Enum"=enum16{"Init", "Log", "Read"}."Log", "state Name"=w1888) -> ()  [unwired: 8 in, 2 out]
          }
          frame condition #1 {
          }
        }
        n780 = call "MB01 Open.vi"() -> ("error out"=w1882:errorcluster)  [unwired: 11 in]
        n781 = Merge Errors(w1878, w1882) -> (w1875:errorcluster)
        n782 = flat-sequence {
          tunnel: [w1887] -> w1876
          tunnel: w1875 -> [w1887]
          frame #0 {
            n783 = Wait (ms)(milliseconds to wait=u32 70) -> ()  [unwired: 1 out]
          }
        }
      }
      frame "INIT.Open COM EMIC" {
        n784 = disable-structure shown="LOGGING==TRUE" {
          disable-tunnel: w1896 -> [w1909 _]
          frame condition #0 (active) {
            n785 = Empty String/Path?(string/path=w1909) -> (empty?=w1912:bool)
            n786 = Select(t="Quece timeout", s=w1912, f=w1909) -> (s? t:f=w1908:string)
            n787 = call "string log (SubVI).vi"("Enum"=enum16{"Init", "Log", "Read"}."Log", "state Name"=w1908) -> ()  [unwired: 8 in, 2 out]
          }
          frame condition #1 {
          }
        }
        n788 = call "Connect to CE14.vi"("Module ID"=-1) -> ("error out"=w1901:errorcluster)  [unwired: 10 in]
        n789 = Merge Errors(w1897, w1901) -> (w1894:errorcluster)
        n790 = flat-sequence {
          tunnel: [w1907] -> w1895
          tunnel: w1894 -> [w1907]
          frame #0 {
            n791 = Wait (ms)(milliseconds to wait=u32 70) -> ()  [unwired: 1 out]
          }
        }
      }
      frame "MEAS.Read EMIC connected" {
        n792 = disable-structure shown="LOGGING==TRUE" {
          disable-tunnel: w1929 -> [w1947 _]
          frame condition #0 (active) {
            n793 = Empty String/Path?(string/path=w1947) -> (empty?=w1950:bool)
            n794 = Select(t="Quece timeout", s=w1950, f=w1947) -> (s? t:f=w1946:string)
            n795 = call "string log (SubVI).vi"("Enum"=enum16{"Init", "Log", "Read"}."Log", "state Name"=w1946) -> ()  [unwired: 8 in, 2 out]
          }
          frame condition #1 {
          }
        }
        n796 = local read "CE14  Module did it"() -> (w1915:bool[])
        n797 = for {
          N: 6 -> [_]
          tunnel: [w1953] -> w1928 mode=indexing
          tunnel: [w1952] -> w1933 mode=indexing
          i -> [w1955]
          n798 = Increment(x=w1955) -> (x+1=w1954:i32)
          n799 = Wait (ms)(milliseconds to wait=u32 50) -> ()  [unwired: 1 out]
          n800 = call "CE14.CheckConnected.vi"("Module ID"=w1954) -> ("error out"=w1952:errorcluster, "Success"=w1953:bool)  [unwired: 8 in, 1 out]
        }
        "EMIC connected" <- w1928
        n801 = And(x=w1915, y=w1928) -> (x .and. y?=w1918:bool[])
        n802 = Index Array(array=w1918) -> (element #1=→"Inst. 4":bool, element #2=→"Inst. 5":bool, element #3=→"Inst. 6":bool, element #4=→"Inst. 7":bool, element #5=→"Inst. 8":bool, element #6=→"Inst. 9":bool)  [unwired: 6 in]
        n803 = Merge Errors(w1932, w1933) -> (w1920:errorcluster)
        n804 = for {
          tunnel: w1918 -> [w1943] mode=indexing
          tunnel: [w1942] -> w1917
          n805 = call "FGV Init phase.vi"("Boolean"=w1943) -> ("Init Completed?"=w1942:bool)  [unwired: 9 in, 1 out]
        }
        n806 = case shown="False" w1917 {
          tunnel: w1916 -> [_ w1941]
          tunnel: [_ w1939] -> w1913
          frame False {
          }
          frame True {
            n807 = call "App enquece.vi"("command"="INIT.Read DRV code", "queue in"=w1941) -> ("error out"=w1939:errorcluster)  [unwired: 8 in, 1 out]
          }
        }
        n808 = Merge Errors(w1920, w1913) -> (w1914:errorcluster)
        n809 = flat-sequence {
          tunnel: [w1944] -> w1921
          tunnel: w1914 -> [w1944]
          frame #0 {
            n810 = Wait (ms)(milliseconds to wait=u32 70) -> ()  [unwired: 1 out]
          }
        }
      }
      frame "MEAS.Set DMM config" {
        n811 = disable-structure shown="LOGGING==TRUE" {
          disable-tunnel: w1959 -> [w1978 _]
          frame condition #0 (active) {
            n812 = Empty String/Path?(string/path=w1978) -> (empty?=w1981:bool)
            n813 = Select(t="Quece timeout", s=w1981, f=w1978) -> (s? t:f=w1977:string)
            n814 = call "string log (SubVI).vi"("Enum"=enum16{"Init", "Log", "Read"}."Log", "state Name"=w1977) -> ()  [unwired: 8 in, 2 out]
          }
          frame condition #1 {
          }
        }
        n815 = Variant To Data(type=T19 {"DMM config cluster"={"DCV range"=0.0, "DCI range"=0.0, "Detector Rate"=0}, "mux2-1(DMM I) encode"=enum."DMM I (0.5)"} ("DMM all config"), Variant=w1971) -> (data=w1969:T19)  [unwired: 1 in, 1 out]
        n816 = Unbundle By Name(w1969) -> ("DMM config cluster"=w1968:T20)
        n817 = Unbundle By Name(w1968) -> ("DCV range"=w1967:dbl, "DCI range"=w1966:dbl, "Detector Rate"=w1965:u8)
        n818 = call "config channel.vi"("Detector Rate"=w1965, "DCI range"=w1966, "DCV range"=w1967) -> ("error out"=w1963:errorcluster)  [unwired: 8 in]
        n819 = Merge Errors(w1960, w1963) -> (w1957:errorcluster)
        n820 = flat-sequence {
          tunnel: [w1976] -> w1958
          tunnel: w1957 -> [w1976]
          frame #0 {
            n821 = Wait (ms)(milliseconds to wait=u32 70) -> ()  [unwired: 1 out]
          }
        }
      }
      frame "MEAS.AllRelaysOFF" {
        n822 = disable-structure shown="LOGGING==TRUE" {
          disable-tunnel: w1984 -> [w1995 _]
          frame condition #0 (active) {
            n823 = Empty String/Path?(string/path=w1995) -> (empty?=w1998:bool)
            n824 = Select(t="Quece timeout", s=w1998, f=w1995) -> (s? t:f=w1994:string)
            n825 = call "string log (SubVI).vi"("Enum"=enum16{"Init", "Log", "Read"}."Log", "state Name"=w1994) -> ()  [unwired: 8 in, 2 out]
          }
          frame condition #1 {
          }
        }
        n826 = for {
          N: 5 -> [_]
          tunnel: [w1999] -> w1989 mode=indexing
          i -> [w2001]
          n827 = case shown="4" w2001 {
            tunnel: [w2005 w2006 w2007 w2008 w2009 _] -> w1999
